vi "ListPublicAttributes.vi"(8 "error in (no error)":errorcluster, 11 "SMO in":refnum<class "SMO.lvclass">) -> (0 "error out":errorcluster, 2 "Public Attributes":string[](array[string]), 3 "SMO out":refnum<class "SMO.lvclass">)   [LabVIEW 2021, in "smo.lvlib" / "SMO.lvclass"]
uses:
  SMO.lvclass
  SMO.lvclass/SMO.ctl
  Support/Attribute/Attribute.lvclass
  Definitions/def.SMO/Scope -- Enum.ctl
  Definitions/def.SMO/def.SMO.lvclass
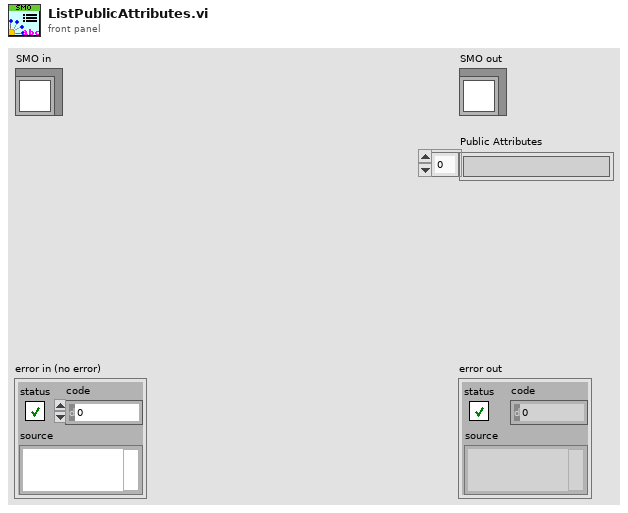
[diagram p1: front panel]
types:
  T1 = typedef "smo.lvlib/def.SMO.lvclass/Scope -- Enum.ctl" = enum16{"Public", "Protected", "Private"}
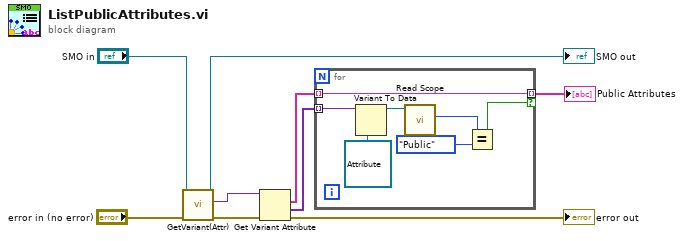
[diagram p0: block diagram]
diagram:
  n1 = call "GetVariant(Attr).vi"("error in (no error)"="error in (no error)", "SMO in"="SMO in") -> ("error out"=w7:errorcluster, "[Attributes]"=w5:variant, "SMO out"=→"SMO out":refnum<class "SMO.lvclass">)  [unwired: 7 in]
  n2 = Get Variant Attribute(Variant=w5, error in=w7) -> (names=w3:string[], values=w4:variant[], error out=→"error out":errorcluster)  [unwired: 2 in, 1 out]
  n3 = for {
    tunnel: w4 -> [w15] mode=indexing
    tunnel: w3 -> [w16] mode=indexing
    tunnel: [w16] -> w2 mode=indexing if=w10
    n4 = Variant To Data(type=refnum<class "Attribute.lvclass"> refnum ("Attribute.lvclass"), Variant=w15) -> (data=w13:refnum<class "Attribute.lvclass">)  [unwired: 1 in, 1 out]
    n5 = call "Read Scope.vi"("Attribute in"=w13) -> ("Scope"=w12:T1)  [unwired: 9 in, 1 out]
    n6 = Equal?(x=w12, y=Scope_--_Enum."Public") -> (x = y?=w10:bool)
  }
  "Public Attributes" <- w2
